vi "event_register_change_out.vi"(8 "error in (no error)":errorcluster) -> (0 "error out":errorcluster, 3 "change_out":refnum<event-registration>)   [LabVIEW 2015, in "lv-recipe-machine.lvlib"]
uses:
  lv-recipe-machine.lvlib
  _controls/change.ctl
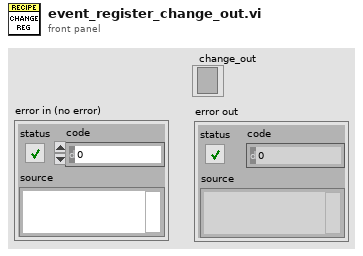
[diagram p1: front panel]
types:
  T1 = typedef "lv-recipe-machine.lvlib/references.ctl" = cluster{"semaphore":T2, "input_queue":refnum<queue>, "output_queue":refnum<queue>, "transition_queue":refnum<queue>, "data_dvr":refnum<data-value>, "stop_notifier":refnum<notifier>, "change_in_event":refnum<user-event>, "change_out_event":refnum<user-event>, "status_event":refnum<user-event>}
  T2 = typedef "Semaphore RefNum" = refnum<k1>
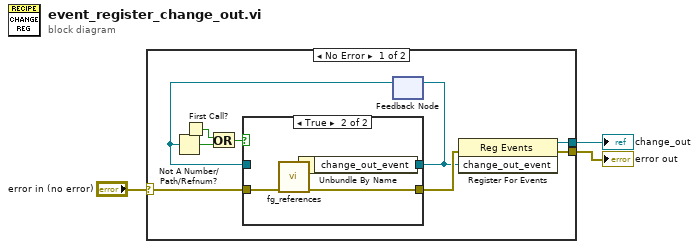
[diagram p0: block diagram]
diagram:
  n1 = case shown="No Error" "error in (no error)" {
    selector: "error in (no error)" -> [w7 w19]
    tunnel: [w5 w19] -> w2
    tunnel: [w4 _] -> w1
    frame No Error {
      n2 = First Call?() -> (First Call?: T/F=w10:bool)
      n3 = feedback #1() -> (w9:refnum<user-event>)  [unwired: 1 in]
      n4 = Not A Number/Path/Refnum?(number/path/refnum=w9) -> (NaN/Path/Refnum?=w11:bool)
      n5 = Or(x=w10, y=w11) -> (x .or. y?=w8:bool)
      n6 = case shown="True" w8 {
        tunnel: w7 -> [w13 w18]
        tunnel: [w13 w17] -> w12
        tunnel: [w14 w15] -> w6
        tunnel: w9 -> [w14 _]
        frame False {
        }
        frame True {
          n7 = call "fg_references.vi"("error in (no error)"=w18) -> ("error out"=w17:errorcluster, "references out"=w16:T1)  [unwired: 9 in]
          n8 = Unbundle By Name(w16) -> ("change_out_event"=w15:refnum<user-event>)
        }
      }
      n9 = feedback-in #1(w6) -> ()
      n10 = register-events(error in=w12, w6) -> (reference out=w4:refnum<event-registration>, error out=w5:errorcluster)  [unwired: 1 in]
    }
    frame Error {
    }
  }
  "error out" <- w2
  "change_out" <- w1
